vi "pcfs_initialize_axis.vi"(8 "error in (no error)":errorcluster, 11 "pcfs in":refnum<class "pcfs.lvclass">) -> (0 "error out":errorcluster, 3 "pcfs out":refnum<class "pcfs.lvclass">)   [LabVIEW 2015, in "pcfs.lvclass"]
uses:
  pcfs.lvclass
  Stage Class/Stage.lvclass
  pcfs.lvclass/pcfs.ctl
  UI/front_panel_class/hardware_caller_queue_numbers.ctl
  UI/panel_class/panel.lvclass
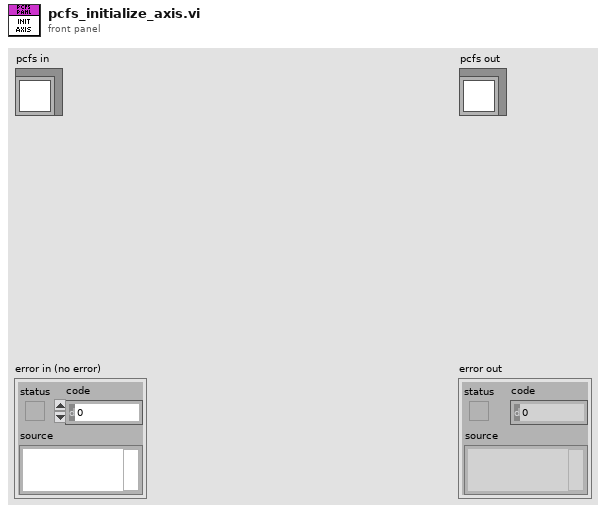
[diagram p1: front panel]
types:
  T1 = typedef "hardware_caller_queue_numbers.ctl" = enum16{"stage1", "stage2", "experiment", "detector"}
  T2 = typedef "pcfs_position_settings.ctl" = cluster{"Center Pos. (mm)":dbl, "increment":dbl, "steps":dbl, "dither_dist":dbl, "dither_period":dbl}
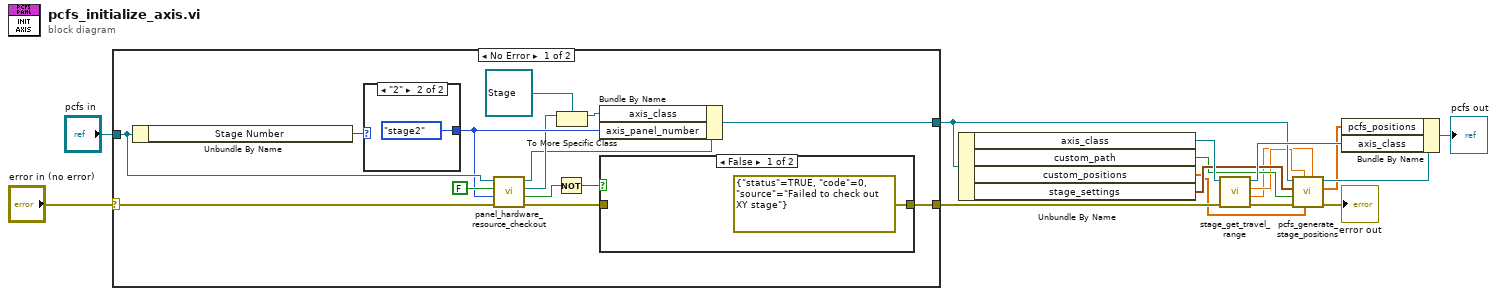
[diagram p0: block diagram]
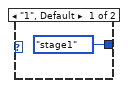
[diagram p3: hidden frame]
diagram:
  n1 = case shown="No Error" "error in (no error)" {
    selector: "error in (no error)" -> [w27 w36]
    tunnel: [w24 w36] -> w9
    tunnel: [w19 w35] -> w7
    tunnel: "pcfs in" -> [w28 w35]
    frame No Error {
      n2 = Unbundle By Name(w28) -> ("Stage Number"=w30:enum16{"1", "2"})
      n3 = case shown="\"2\"" w30 {
        tunnel: [hardware_caller_queue_numbers."stage1" ("panel_number") hardware_caller_queue_numbers."stage2" ("panel_number")] -> w22
        frame "1", Default {
        }
        frame "2" {
        }
      }
      n4 = call "panel_hardware_resource_checkout.vi"("error in (no error)"=w27, "panel_number"=w22, "Self?"=FALSE, "panel in"=w28) -> ("error out"=w17:errorcluster, "timed out?"=w25:bool, "hardware.lvclass"=w21:refnum<class "hardware.lvclass">, "panel out"=w18:refnum<class "pcfs.lvclass">)  [unwired: 4 in]
      n5 = Not(x=w25) -> (.not. x?=w23:bool)
      n6 = To More Specific Class(target class=refnum<class "Stage.lvclass"> refnum ("Stage.lvclass"), reference=w21) -> (specific class reference=w20:refnum<class "Stage.lvclass">)  [unwired: 1 in, 1 out]
      n7 = Bundle By Name(cluster=w18, "axis_class"=w20, "axis_panel_number"=w22) -> (w19:refnum<class "pcfs.lvclass">)
      n8 = case shown="False" w23 {
        tunnel: [errorcluster {"status"=TRUE, "code"=0, "source"="Failed to check out XY stage"} ("error out") w32] -> w24
        tunnel: w17 -> [_ w32]
        frame False {
        }
        frame True {
        }
      }
    }
    frame Error {
    }
  }
  n9 = Unbundle By Name(w7) -> ("axis_class"=w14:refnum<class "Stage.lvclass">, "custom_path"=w5:bool, "custom_positions"=w2:dbl[], "stage_settings"=w8:T2)
  n10 = call-dynamic "stage_get_travel_range.vi"("error in (no error)"=w9, "Stage in"=w14) -> ("error out"=w12:errorcluster, "min(mm)"=w3:dbl, "max (mm)"=w4:dbl, "Stage out"=w13:refnum<class "Stage.lvclass">)  [unwired: 6 in]
  n11 = call "pcfs_generate_stage_positions.vi"("travel_min (mm)"=w3, "custom_positions"=w2, "travel_max (mm)"=w4, "error in (no error)"=w12, "custom_trajectory"=w5, "pcfs_settings"=w8, "scan_panel in"=w7) -> ("error out"=→"error out":errorcluster, "Positions (mm)"=w1:dbl[], "scan_panel out"=w6:refnum<class "pcfs.lvclass">)  [unwired: 2 out]
  n12 = Bundle By Name(cluster=w6, "pcfs_positions"=w1, "axis_class"=w13) -> (→"pcfs out":refnum<class "pcfs.lvclass">)
